vi "离线得到原始码.vi"(8 "错误输入":errorcluster caption="输出簇", 9 "读取字节数":u32, 10 "读取位置":i32, 11 "文件句柄":i32) -> (0 "错误输出":errorcluster, 1 "实际字节数":u32, 2 "原始码":u8[](array[numeric]), 3 "文件句柄出":i32)   [LabVIEW 2011]
uses:
  dll/em9636.dll
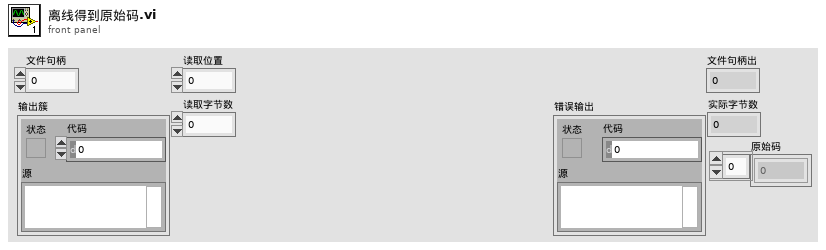
[diagram p1: front panel]
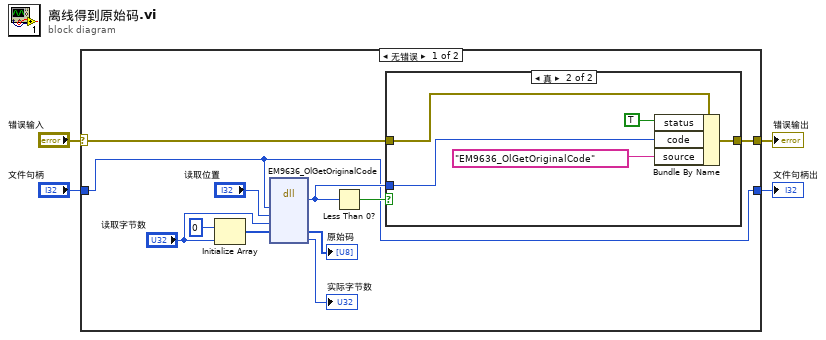
[diagram p0: block diagram]
diagram:
  n1 = case shown="无错误" "错误输入" {
    selector: "错误输入" -> [w11 w23]
    tunnel: [w13 w23] -> w3
    tunnel: "文件句柄" -> [w12 w22]
    tunnel: [w12 w22] -> w1
    frame No Error {
      n2 = Initialize Array(u8 0 ("元素"), "读取字节数") -> (w7:u8[])
      n3 = dll-call lib="PTH1abs Eèµ éç LABVIEWæºVI(v2.0)EM9636BD)EM9636BDè°ç¨APIå½æ°æ¹æ³éè®¯ä¾ç¨EM9636labview8.5-1511048.5dll\nem9636.dll" fn="EM9636_OlGetOriginalCode"("文件句柄"=w12, "读取位置"="读取位置", "读取字节数"="读取字节数", "原始码"=w7) -> ("错误信息"=w14:i32, "原始码"=→"原始码":u8[], "实际字节数"=→"实际字节数":u32)  [unwired: 7 in, 2 out]
      n4 = Less Than 0?(x=w14) -> (x < 0?=w15:bool)
      n5 = case shown="真" w15 {
        tunnel: [w16 w19] -> w13
        tunnel: w11 -> [w16 w21]
        tunnel: w14 -> [_ w18]
        frame False {
        }
        frame True {
          n6 = Bundle By Name(cluster=w21, "status"=TRUE, "code"=w18, "source"="EM9636_OlGetOriginalCode") -> (w19:errorcluster)
        }
      }
    }
    frame Error {
    }
  }
  "文件句柄出" <- w1
  "错误输出" <- w3
